vi "Clear Component Lists.vi"(8 "error in (no error)":errorcluster, 11 "MLA in":refnum<class "MLA.lvclass">) -> (0 "error out":errorcluster, 3 "MLA out":refnum<class "MLA.lvclass">)   [LabVIEW 2023]
uses:
  MLA/MLA.lvclass
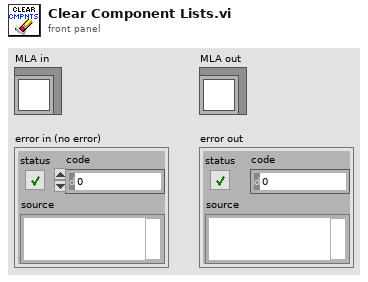
[diagram p1: front panel]
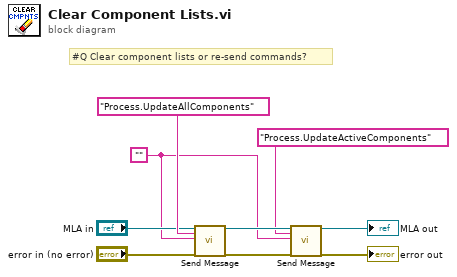
[diagram p0: block diagram]
diagram:
  w1 = ""
  # "#Q Clear component lists or re-send commands?"
  n1 = call-dynamic "Send Message.vi"("MLA"="MLA in", "Message"="Process.UpdateAllComponents", "Param 1"=w1, "error in (no error)"="error in (no error)") -> ("MLA"=w4:refnum<class "MLA.lvclass">, "error out"=w7:errorcluster)  [unwired: 14 in]
  n2 = call-dynamic "Send Message.vi"("MLA"=w4, "Message"="Process.UpdateActiveComponents", "Param 1"=w1, "error in (no error)"=w7) -> ("MLA"=→"MLA out":refnum<class "MLA.lvclass">, "error out"=→"error out":errorcluster)  [unwired: 14 in]
